vi "GetRFFrame.vi"() -> ()   [LabVIEW 2022 SP3]
uses:
  Motion Controllers/-MotionRoutines/MotionGlobals.vi
  <instrlib>/vi.lib/Platform/portaccess.llb/Out Port32.vi
  <instrlib>/Acqiris Dx/Acqiris Dx.lvlib
  <instrlib>/Acqiris Bx/Acqiris Bx.lvlib
  <instrlib>/niScope/Acquire/Fetch/niScope Multi Fetch Binary 8.vi
  <vilib>/Platform/TimedLoop/XDataNode/XDataNode.xnode
  <vilib>/Platform/TimedLoop/XDataNode/nitl_modes.ctl
  <vilib>/Platform/TimedLoop/XDataNode/XDNodeRunTimeDep.lvlib
  <vilib>/Platform/TimedLoop/XDataNode/wakeup.ctl
  <vilib>/Platform/TimedLoop/XDataNode/timing_clust.ctl
  Pulsers/pulser.ctl
  Acqiris/-AcqirisRoutines/VScaleInfoAcq.vi
panel:
  in  "power":u16(ring)=1 items=["1"=1, "2"=2, "3"=3, "4"=4, "5"=5, "6"=6, "7"=7, "8"=8, "9"=9, "10"=10, "20"=20, "30"=30, "40"=40, "50"=50, "60"=60, "70"=70, "80"=80, "90"=90, "100"=100]
  out "RealFileName":string
  in  "View EYE":bool
  in  "Acq mode":T1(tab)
  in  "Get Frame":bool
  in  "Autosave?":bool
  in  "Save Single":bool
  in  "Reverse Off":bool
  in  "Cont Frame":bool
  in  "Frame Divide":u32=1 min=1
  in  "Fixed Frame Delay":bool
  in  "frame time (ms)":u32=100 min=1
  out "Loop Time":u64=1000
  in  "Total Time (s)":u32=10 min=1
  out "Frame":i32
  in  "Dummy V":dbl
  out "Memory Size (Byte)":i32 format="%^.0e"
  in  "Data Path":path=path "F:/Temp"
  in  "Num of Frames":i32=1
  in  "Set up Dig":bool
  in  "RF cycles":i16=1 min=1
  in  "Display?":bool=TRUE
  in  "ResetNumbing":bool
  in  "file name":string
  out "subarray":i16[][](array[numeric])
  out "Raw data":dbl[][](graph)
  out "Att (dB)":sgl format="%#_1f"
  in  "stop":bool
  in  "Num of Vectors":i32=464
  # "Vevo 770 #s (for header and file name)"
  # "0 dB would scale data to 1 Vpp. 20 dB to 10 Vpp, etc."
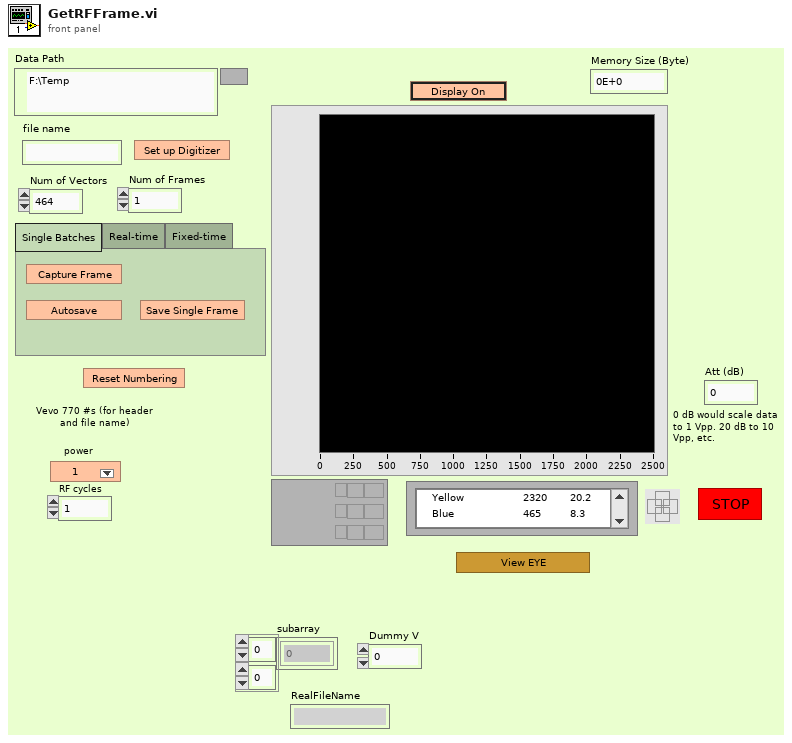
[diagram p1: front panel]
types:
  T1 = enum32{"Single Batches", "Real-time", "Fixed-time"}
  T2 = typedef "pulser.ctl" = enum16{"Pan 5900", "Agilent 33250A", "WMC Mono-Cycle", "Blank", "NYU AVTECH", "Tabor W1281A", "Daxsonics BP1", "Pan 5800", "Daxsonics BP2"}
  T3 = typedef "XDNodeRunTimeDep.lvlib/timing_clust.ctl" = cluster{"Expected End [f-1]":u64, "Actual End [f-1]":u64, "Finished Late? [f-1]":bool, "Expected End [i-1]":u64, "Actual End [i-1]":u64, "Finished Late? [i-1]":bool, "Expected Start [i]":u64, "Actual Start [i]":u64, "Expected Start [f]":u64, "Actual Start [f]":u64, "Source Name":string, "Structure Name":string, "Period":i64, "Deadline":i64, "Offset":i64, "Start":i64, "Priority":i32, "Timeout":i32, "Mode":T4, "Wakeup Reason":T5, "Error":errorcluster, "Source Type":string, "Secondary Source Type":string, "Global End Time":u64, "Global Start Time":u64, "Frame Duration":u64, "Iteration Duration":u64, "Assigned CPU":i32, "I/O Scan Engine Mode":u32}
  T4 = typedef "XDNodeRunTimeDep.lvlib/nitl_modes.ctl" = enum32{"No Change", "Process missed periods, maintain original phase", "Discard missed periods, maintain original phase", "Process missed periods, ignore original phase", "Discard missed periods, ignore original phase"}
  T5 = typedef "XDNodeRunTimeDep.lvlib/wakeup.ctl" = enum32{"Normal", "Aborted", "Asynchronous wakeup", "Timing source error", "Timed loop error", "Timeout"}
  T6 = cluster{"Sampling Rate":dbl, "Ref Delay (ms)":dbl, "rf points per line":i32}
  T7 = cluster{sgl, "Gain [dB]  ":sgl, "Atten (dB)":sgl}
  T8 = cluster{"actualSamples":i32, "absoluteInitialX":dbl, "relativeInitialX":dbl, "xIncrement":dbl, "offset":dbl, "gain":dbl, "reserved1":dbl, "reserved2":dbl}[]
  T9 = cluster{"actualSamples":i32, "absoluteInitialX":dbl, "relativeInitialX":dbl, "xIncrement":dbl, "offset":dbl, "gain":dbl, "reserved1":dbl, "reserved2":dbl}
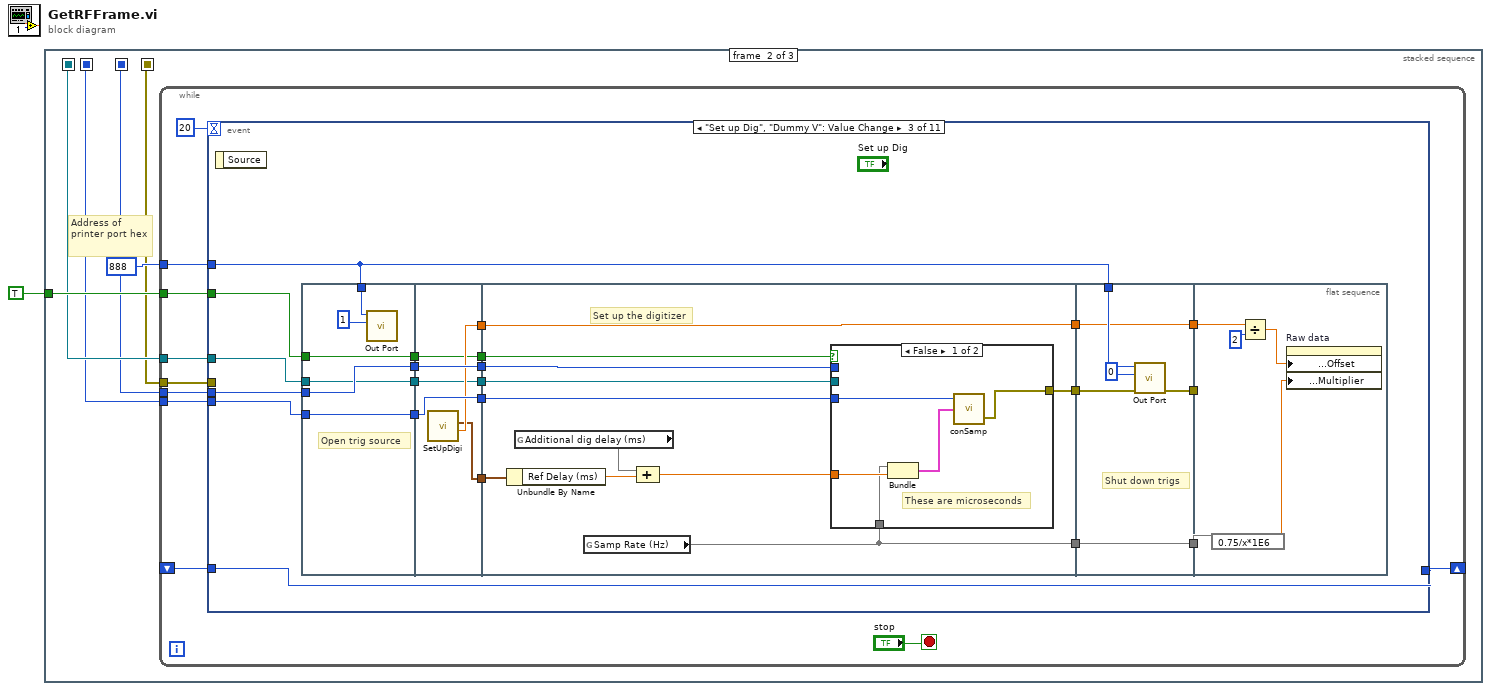
[diagram p0: block diagram]
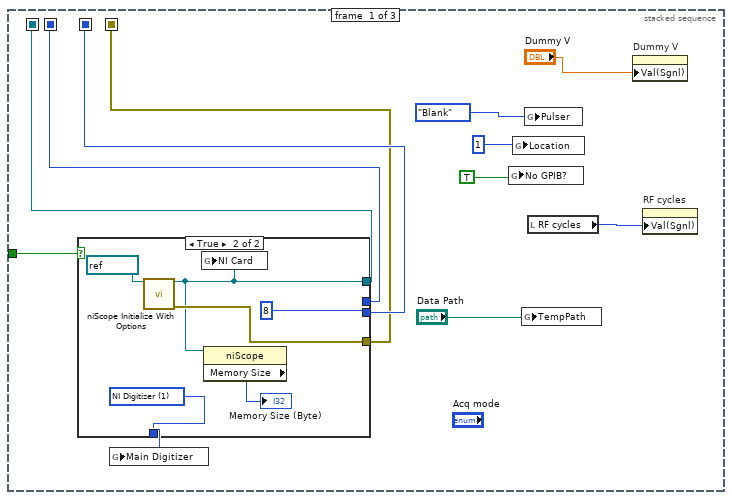
[diagram p2: hidden frame]
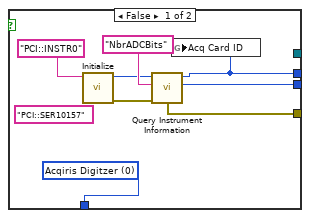
[diagram p3: hidden frame]
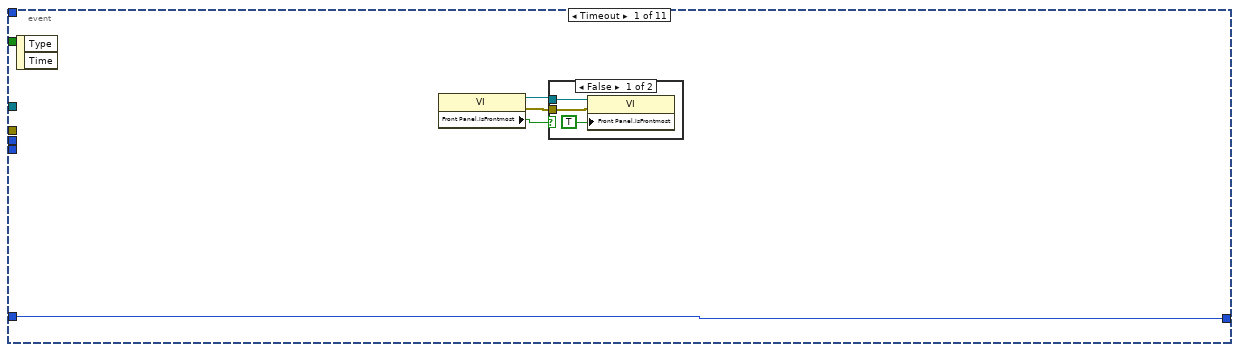
[diagram p4: hidden frame]
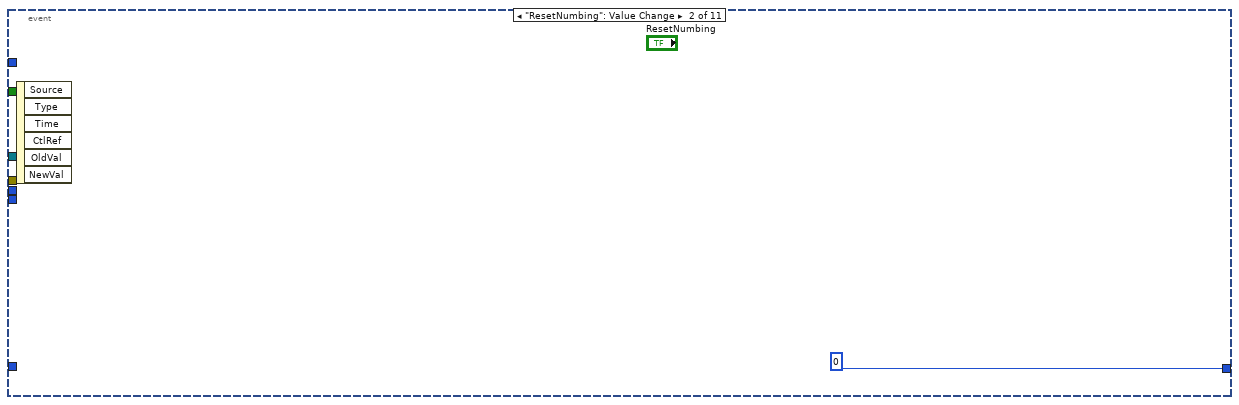
[diagram p6: hidden frame]
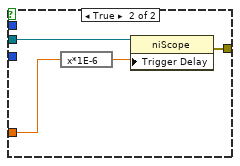
[diagram p7: hidden frame]
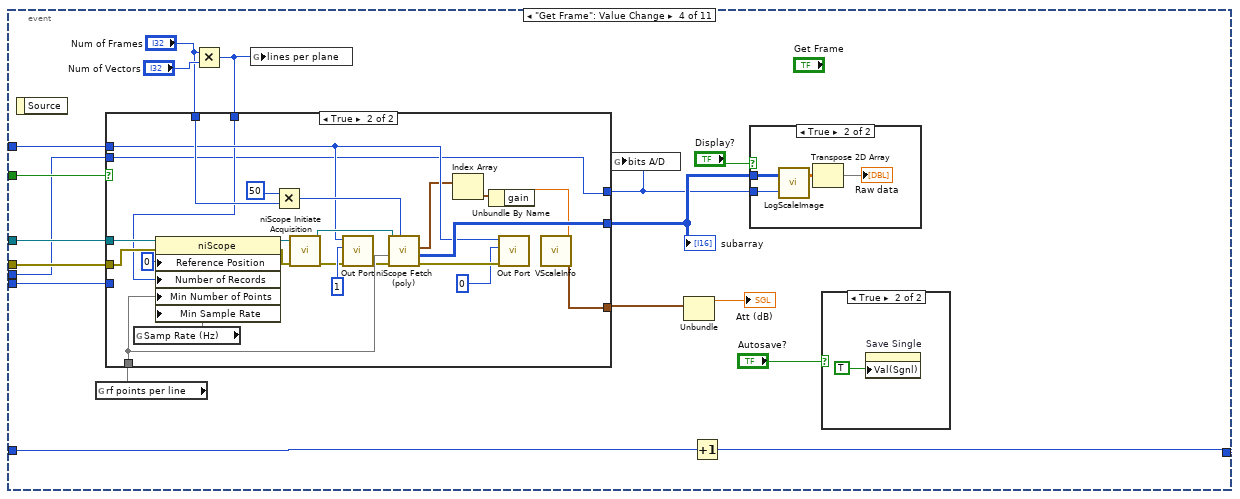
[diagram p8: hidden frame]
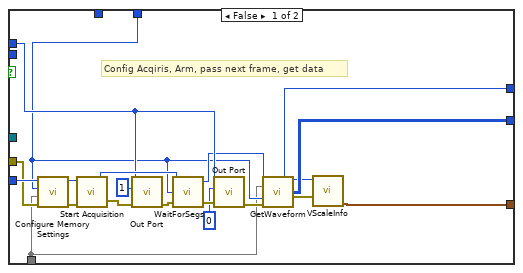
[diagram p9: hidden frame]
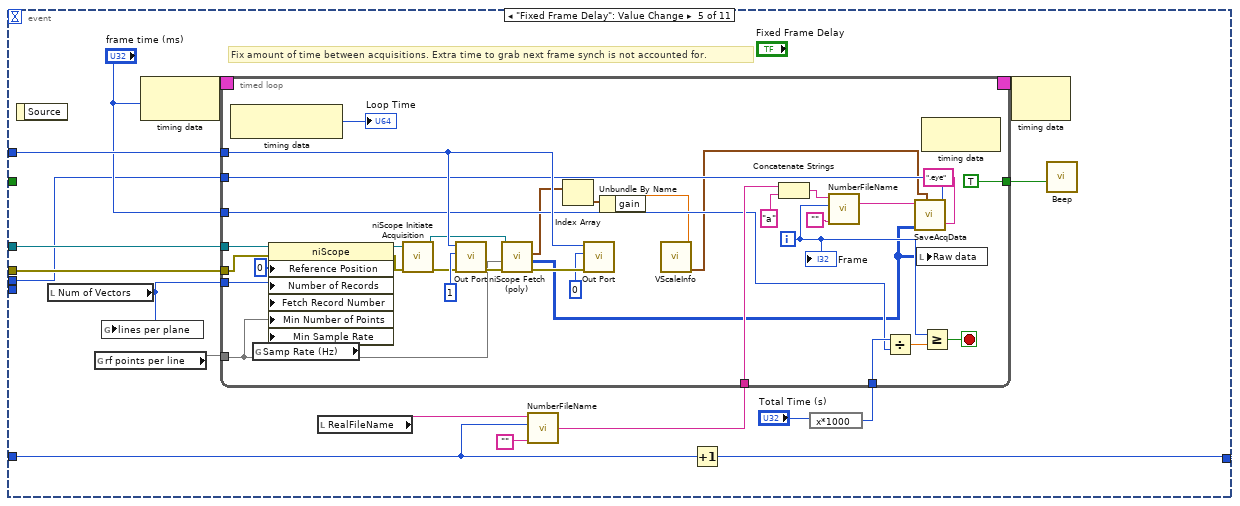
[diagram p12: hidden frame]
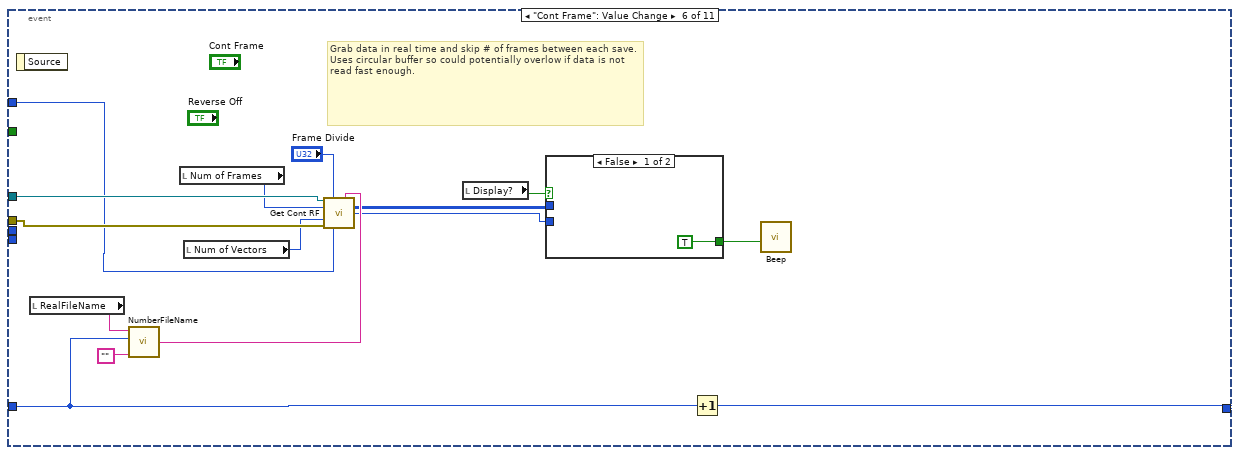
[diagram p13: hidden frame]
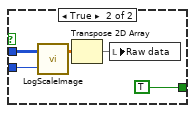
[diagram p14: hidden frame]
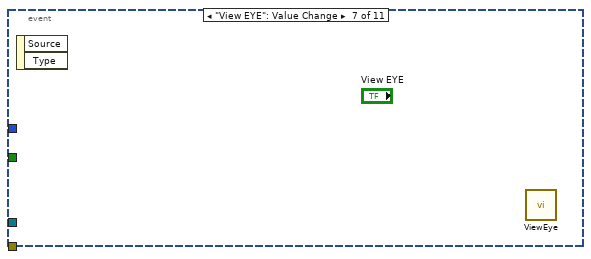
[diagram p15: hidden frame]
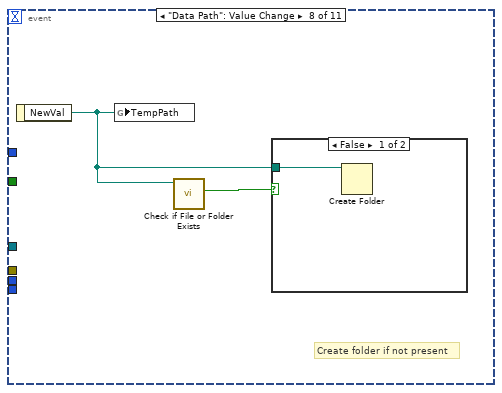
[diagram p16: hidden frame]
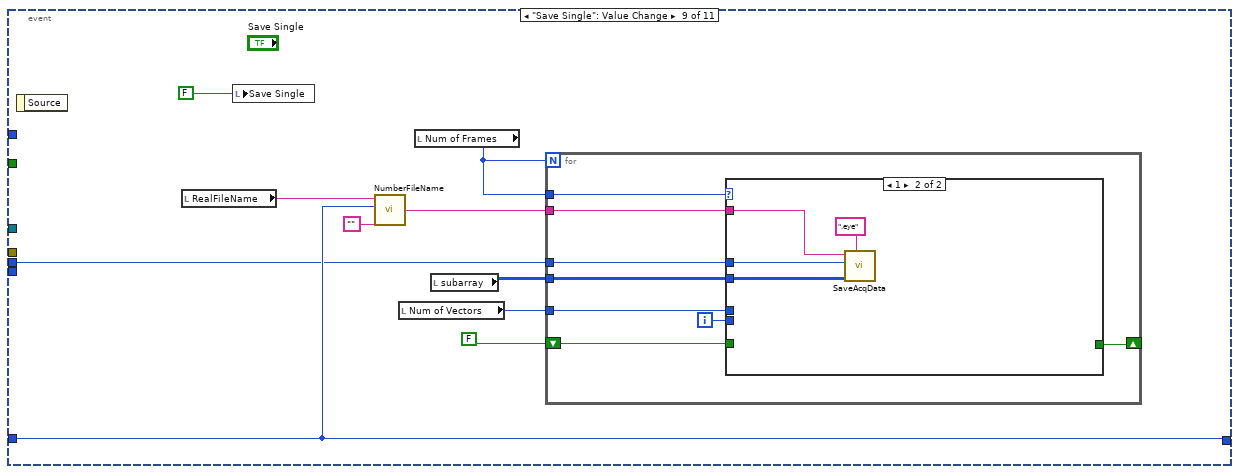
[diagram p18: hidden frame]
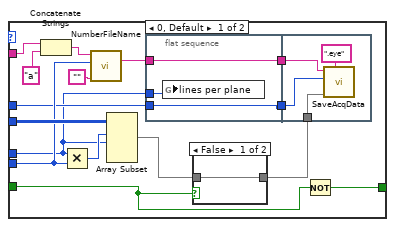
[diagram p19: hidden frame]
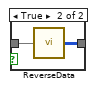
[diagram p20: hidden frame]
diagram:
  n1 = stacked-sequence {
    seq-local: [w9 _ _] -> [_ w31 w320]
    seq-local: [w8 _ _] -> [_ w30 _]
    seq-local: [w7 _ _] -> [_ w29 _]
    seq-local: [w6 _ _] -> [_ w28 _]
    tunnel: TRUE -> [w10 w32 w319]
    frame #0 {
      n2 = case shown="True" w10 {
        tunnel: [_ w24] -> w9
        tunnel: [w18 w25] -> w6
        tunnel: [w14 _] -> w8
        tunnel: [w17 8] -> w7
        tunnel: [w15 w22] -> w11
        frame False {
          w15 = u16 0 items=["Acqiris Digitzer", "NI Digitizer"] ("Main Digitizer")
          (unwired) "PCI::SER10157" ("ResourceName")
          n3 = call <instrlib>:"Initialize.vi"("Resource Name (PCI::INSTR0)"="PCI::INSTR0" ("ResourceName")) -> ("error out"=w19:errorcluster, "Instrument ID"=w20:u32)  [unwired: 3 in, 2 out]
          n4 = call <instrlib>:"Query Instrument Information.vi"("Instrument ID"=w20, "Parameter String"="NbrADCBits", "error in (no error)"=w19) -> ("dup Instrument ID"=w14:u32, "Info Value (I32)"=w17:i32, "error out"=w18:errorcluster)  [unwired: 1 in, 3 out]
          n5 = global write "MotionGlobals.vi" "Acq Card ID"(w14) -> ()
        }
        frame True {
          w22 = u16 1 items=["Acqiris Digitzer", "NI Digitizer"] ("Main Digitizer")
          n6 = call <instrlib>:"niScope Initialize With Options.vi"("resource name"=refnum<k15> "Dig1") -> ("instrument handle"=w24:refnum<k15>, "error out"=w25:errorcluster)  [unwired: 4 in, 9 out]
          n7 = global write "MotionGlobals.vi" "NI Card"(w24) -> ()
          n8 = property class="niScope"(reference=w24) -> ("Memory Size"=→"Memory Size (Byte)":i32)  [unwired: 1 in, 2 out]
        }
      }
      n9 = global write "MotionGlobals.vi" "Main Digitizer"(w11) -> ()
      n10 = global write "MotionGlobals.vi" "No GPIB?"(TRUE ("No GPIB?")) -> ()
      n11 = global write "MotionGlobals.vi" "Location"(1) -> ()
      n12 = global write "MotionGlobals.vi" "TempPath"("Data Path") -> ()
      n13 = global write "MotionGlobals.vi" "Pulser"(pulser."Blank" ("Pulser")) -> ()
      n14 = local read "RF cycles"() -> (w2:i16)
      n15 = property on="Dummy V" class="DigNum (strict)"("Val(Sgnl)"="Dummy V") -> ()  [unwired: 2 in, 2 out]
      n16 = property on="RF cycles" class="DigNum (strict)"("Val(Sgnl)"=w2) -> ()  [unwired: 2 in, 2 out]
    }
    frame #1 {
      # "Address of printer port hex"
      n17 = while {
        tunnel: w31 -> [w43]
        shift-right: [w39] -> _
        shift-left: _ -> [w40]
        tunnel: w30 -> [w38]
        tunnel: w32 -> [w37]
        tunnel: w28 -> [w36]
        tunnel: i16 888 ("address") -> [w35]
        tunnel: w29 -> [w34]
        stop <- "stop" stop-if-true
        n18 = event shown="[2] \"Set up Dig\", \"Dummy V\": Value Change" {
          selector: _ -> [_ _ _ _ _ _ _ _ _ _ _]
          dyn-events: _ -> [_ _ _ _ _ _ _ _ _ _ _]
          timeout: 20 -> [_ _ _ _ _ _ _ _ _ _ _]
          tunnel: w43 -> [_ _ w57 w134 w200 w256 _ _ _ _ _]
          tunnel: w36 -> [_ _ _ w133 w199 w255 _ _ _ _ _]
          tunnel: w40 -> [w47 _ w61 w129 w191 w248 _ _ w275 _ _]
          tunnel: [w47 0 w61 w128 w197 w254 _ _ w275 _ _] -> w39
          tunnel: w38 -> [_ _ w73 w131 _ _ _ _ _ _ _]
          tunnel: w37 -> [_ _ w60 w132 _ _ _ _ _ _ _]
          tunnel: w35 -> [_ _ w72 w130 w198 w251 _ _ _ _ _]
          tunnel: w34 -> [_ _ w71 w117 w184 _ _ _ w274 _ _]
          event Timeout {
            n19 = event-data() -> ()  [unwired: 3 out]
            n20 = property class="VI"() -> (reference out=w46:refnum<vi>, error out=w45:errorcluster, "Front Panel.IsFrontmost"=w44:bool)  [unwired: 2 in]
            n21 = case shown="False" w44 {
              tunnel: w46 -> [w50 _]
              tunnel: w45 -> [w48 _]
              frame False {
                n22 = property class="VI"(reference=w50, error in=w48, "Front Panel.IsFrontmost"=TRUE) -> ()  [unwired: 2 out]
              }
              frame True {
              }
            }
          }
          event "ResetNumbing": Value Change {
            n23 = event-data() -> ()  [unwired: 7 out]
          }
          event "Set up Dig", "Dummy V": Value Change {
            n24 = event-data() -> ()  [unwired: 2 out]
            n25 = flat-sequence {
              tunnel: w73 -> [w79]
              tunnel: [w79] -> w70
              tunnel: w72 -> [w77]
              tunnel: [w76] -> w68
              tunnel: w71 -> [w76]
              tunnel: w60 -> [w75]
              tunnel: [w75] -> w58
              tunnel: w57 -> [w74]
              tunnel: [w74] -> w55
              tunnel: w70 -> [w84]
              tunnel: [w84] -> w69
              tunnel: w68 -> [w85]
              tunnel: [w85] -> w67
              tunnel: [w83] -> w62
              tunnel: [w82] -> w59
              tunnel: w58 -> [w82]
              tunnel: [w81] -> w56
              tunnel: w55 -> [w81]
              tunnel: [w80] -> w54
              tunnel: w69 -> [w96]
              tunnel: w67 -> [w95]
              tunnel: [w87] -> w65
              tunnel: [w86] -> w63
              tunnel: w62 -> [w86]
              tunnel: w59 -> [w94]
              tunnel: w56 -> [w93]
              tunnel: w54 -> [w92]
              tunnel: [w88] -> w53
              tunnel: w72 -> [w110]
              tunnel: [w109] -> w66
              tunnel: w65 -> [w109]
              tunnel: [w108] -> w64
              tunnel: w63 -> [w108]
              tunnel: w53 -> [w107]
              tunnel: [w106] -> w52
              tunnel: w66 -> [w116]
              tunnel: w64 -> [w113]
              tunnel: w52 -> [_]
              frame #0 {
                # "Open trig source"
                n26 = call-poly <instrlib>:"Out Port.vi"("write value"=1, "address"=w77) -> ()  [unwired: 1 in, 7 out]
              }
              frame #1 {
                n27 = call "SetUpDigi.vi"() -> ("Equivalent RT delay\ndistance (mm)"=w83:dbl, "RF data Sampling Out"=w80:T6)  [unwired: 5 in, 5 out]
              }
              frame #2 {
                # "Set up the digitizer"
                n28 = Unbundle By Name(w92) -> ("Ref Delay (ms)"=w90:dbl)
                n29 = global read "MotionGlobals.vi" "Additional dig delay (ms)"() -> (w91)
                n30 = global read "MotionGlobals.vi" "Samp Rate (Hz)"() -> (w87)
                n31 = Compound Arithmetic op=ADD(w91, w90) -> (w89:dbl)
                n32 = case shown="False" w94 {
                  tunnel: w96 -> [w98 _]
                  tunnel: w95 -> [_ _]
                  tunnel: w93 -> [_ w102]
                  tunnel: w89 -> [w101 w104]
                  tunnel: [w99 w103] -> w88
                  tunnel: w87 -> [w97 _]
                  frame False {
                    # "These are microseconds"
                    n33 = Bundle("Samp Rate (Hz)"=w97, w101) -> (w100:cluster{"Samp Rate (Hz)":void, dbl})  [unwired: 1 out]
                    n34 = call "conSamp.vi"("Sampling"=w100, "InstrumentID"=w98) -> ("error out"=w99:errorcluster)  [unwired: 1 in, 1 out]
                  }
                  frame True {
                    n35 = expression code="x*1E-6"(w104) -> (w105:dbl)
                    n36 = property class="niScope"(reference=w102, "Trigger Delay"=w105) -> (error out=w103:errorcluster)  [unwired: 1 in, 1 out]
                  }
                }
              }
              frame #3 {
                # "Shut down trigs"
                n37 = call-poly <instrlib>:"Out Port.vi"("error in (no error)"=w107, "write value"=0, "address"=w110) -> ("error out"=w106:errorcluster)  [unwired: 6 out]
              }
              frame #4 {
                n38 = expression code="0.75/x*1E6"(w116) -> (w115:dbl)
                n39 = Divide(x=w113, y=2) -> (x/y=w112:dbl)
                n40 = property on="Raw data" class="IntGraph (strict)"("Y Scale.Offset and Multiplier:Offset"=w112, "Y Scale.Offset and Multiplier:Multiplier"=w115) -> ()  [unwired: 2 in, 2 out]
              }
            }
          }
          event "Get Frame": Value Change {
            n41 = event-data() -> ()  [unwired: 2 out]
            n42 = global read "MotionGlobals.vi" "rf points per line"() -> (w125)
            n43 = Multiply(x="Num of Frames", y="Num of Vectors") -> (x*y=w124:i32)
            n44 = case shown="True" w132 {
              tunnel: w134 -> [_ w173]
              tunnel: w133 -> [w151 w172]
              tunnel: [w142 w177] -> w121
              tunnel: [w137 w158] -> w119
              tunnel: w131 -> [w154 _]
              tunnel: w130 -> [w146 w163]
              tunnel: w124 -> [w136 w161]
              tunnel: w125 -> [w135 w171]
              tunnel: [w143 w176] -> w118
              tunnel: "Num of Frames" -> [_ w168]
              tunnel: w117 -> [_ w158]
              frame False {
                # "Config Acqiris, Arm, pass next frame, get data"
                n45 = call <instrlib>:"Configure Memory Settings.vi"("error in (no error)"=w151, "Number of Samples (1000)"=w135, "Number of Segments (1)"=w136, "Instrument ID"=w154) -> ("error out"=w152:errorcluster, "dup Instrument ID"=w153:u32)  [unwired: 2 out]
                n46 = call <instrlib>:"Start Acquisition.vi"("error in (no error)"=w152, "Instrument ID"=w153) -> ("error out"=w148:errorcluster, "dup Instrument ID"=w150:u32)  [unwired: 2 in]
                n47 = call-poly <instrlib>:"Out Port.vi"("error in (no error)"=w148, "write value"=1, "address"=w146) -> ("error out"=w147:errorcluster)  [unwired: 6 out]
                n48 = call "WaitForSegs.vi"("Acqiris ID"=w150, "lines per plane"=w136, "error in"=w147) -> ("dup Instrument ID"=w141:u32, "error out"=w149:errorcluster)  [unwired: 1 in, 2 out]
                n49 = call-poly <instrlib>:"Out Port.vi"("error in (no error)"=w149, "write value"=0, "address"=w146) -> ("error out"=w138:errorcluster)  [unwired: 6 out]
                n50 = call "GetWaveform.vi"("Acq ID Out"=w141, "Num Samps"=w135, "Num Segs"=w136, "error in"=w138) -> ("Dig Word Size"=w137:u16, "Acq ID Out"=w140:u32, "Acquired Waveform16 bit"=w142:i16[][], "error out"=w139:errorcluster)  [unwired: 2 in, 6 out]
                n51 = call-poly "VScaleInfo.vi"(4:w139, "vGain scalar"=w140) -> ("Voltage Scale"=w143:T7)  [unwired: 6 in, 2 out]
              }
              frame True {
                n52 = global read "MotionGlobals.vi" "Samp Rate (Hz)"() -> (w159)
                n53 = property class="niScope"(reference=w173, error in=w172, "Reference Position"=0, "Number of Records"=w161, "Min Number of Points"=w171, "Min Sample Rate"=w159) -> (reference out=w175:refnum<k15>, error out=w174:errorcluster)
                n54 = Multiply(x=50, y=w168) -> (x*y=w169:i32)
                n55 = call <instrlib>:"niScope Initiate Acquisition.vi"("instrument handle"=w175, "error in"=w174) -> ("instrument handle out"=w178:refnum<k15>, "error out"=w166:errorcluster)  [unwired: 12 out]
                n56 = call-poly <instrlib>:"Out Port.vi"("error in (no error)"=w166, "write value"=1, "address"=w163) -> ("error out"=w165:errorcluster)  [unwired: 6 out]
                n57 = call-poly <instrlib>:"niScope Fetch (poly).vi"("timeout"=w169, "error in"=w165, "numSamples"=w171, "instrument handle"=w178) -> ("error out"=w164:errorcluster, "wfm"=w177:i8[][], "wfm info"=w157:T8)  [unwired: 1 in, 4 out]
                n58 = Index Array(array=w157) -> (element=w156:T9)  [unwired: 1 in]
                n59 = Unbundle By Name(w156) -> ("gain"=w155:dbl)
                n60 = call-poly <instrlib>:"Out Port.vi"("error in (no error)"=w164, "write value"=0, "address"=w163) -> ()  [unwired: 7 out]
                n61 = call-poly "VScaleInfo.vi"("vGain scalar"=w155) -> ("Voltage Scale"=w176:T7)  [unwired: 7 in, 2 out]
              }
            }
            "subarray" <- w121
            n62 = global write "MotionGlobals.vi" "lines per plane"(w124) -> ()
            n63 = global write "MotionGlobals.vi" "bits A/D"(w119) -> ()
            n64 = Unbundle(w118) -> (→"Att (dB)":sgl)  [unwired: 2 out]
            n65 = Increment(x=w129) -> (x+1=w128:i32)
            n66 = case shown="True" "Display?" {
              tunnel: w121 -> [_ w182]
              tunnel: w119 -> [_ w180]
              frame False {
              }
              frame True {
                n67 = call "LogScaleImage.vi"("A/D bits"=w180, "input array"=w182) -> ("log scale image"=w181:dbl[][])  [unwired: 1 out]
                n68 = Transpose 2D Array(2D array=w181) -> (transposed array=→"Raw data":dbl[][])
              }
            }
            n69 = case shown="True" "Autosave?" {
              frame False {
              }
              frame True {
                n70 = property on="Save Single" class="Bool (strict)"("Val(Sgnl)"=TRUE ("Value (Signaling)")) -> ()  [unwired: 2 in, 2 out]
              }
            }
          }
          event "Fixed Frame Delay": Value Change {
            # "Fix amount of time between acquisitions. Extra time to grab next frame synch is not accounted for."
            n71 = event-data() -> ()  [unwired: 2 out]
            n72 = local read "Num of Vectors"() -> (w195:i32)
            n73 = global read "MotionGlobals.vi" "rf points per line"() -> (w196)
            n74 = global write "MotionGlobals.vi" "lines per plane"(w195) -> ()
            n75 = node-c288("frame time (ms)") -> (w194:T3)
            n76 = local read "RealFileName"() -> (w192:string)
            n77 = call "NumberFileName.vi"("String"="", "File number"=w191, "file name"=w192) -> ("Numbered File"=w189:string)  [unwired: 1 in]
            n78 = Increment(x=w191) -> (x+1=w197:i32)
            n79 = expression code="x*1000"("Total Time (s)") -> (w187:u32)
            n80 = timed-loop {
              timing: w194 -> [_]
              timing-out: [_] -> w193
              tunnel: w200 -> [w234]
              tunnel: w199 -> [w233]
              tunnel: w198 -> [w232]
              tunnel: w196 -> [w214]
              tunnel: w195 -> [w222]
              tunnel: w189 -> [w217]
              tunnel: w187 -> [w213]
              tunnel: "frame time (ms)" -> [w212]
              tunnel: [TRUE] -> w185
              tunnel: w184 -> [w205]
              i -> [w211]
              stop <- w209 stop-if-true
              w208 = 0
              n81 = node-c288() -> (→"Loop Time":i64)  [unwired: 1 out]
              n82 = global read "MotionGlobals.vi" "Samp Rate (Hz)"() -> (w223)
              n83 = property class="niScope"(reference=w234, error in=w233, "Reference Position"=w208, "Number of Records"=w222, "Fetch Record Number"=w208, "Min Number of Points"=w214, "Min Sample Rate"=w223) -> (reference out=w230:refnum<k15>, error out=w229:errorcluster)
              n84 = call <instrlib>:"niScope Initiate Acquisition.vi"("instrument handle"=w230, "error in"=w229) -> ("instrument handle out"=w231:refnum<k15>, "error out"=w227:errorcluster)  [unwired: 12 out]
              n85 = call-poly <instrlib>:"Out Port.vi"("error in (no error)"=w227, "write value"=1, "address"=w232) -> ("error out"=w226:errorcluster)  [unwired: 6 out]
              n86 = call-poly <instrlib>:"niScope Fetch (poly).vi"("error in"=w226, "numSamples"=w214, "instrument handle"=w231) -> ("error out"=w225:errorcluster, "wfm"=w207:i8[][], "wfm info"=w203:T8)  [unwired: 2 in, 4 out]
              n87 = Index Array(array=w203) -> (element=w202:T9)  [unwired: 1 in]
              n88 = call-poly <instrlib>:"Out Port.vi"("error in (no error)"=w225, "write value"=0, "address"=w232) -> ()  [unwired: 7 out]
              n89 = Unbundle By Name(w202) -> ("gain"=w201:dbl)
              n90 = call-poly "VScaleInfo.vi"("vGain scalar"=w201) -> ("Voltage Scale"=w204:T7)  [unwired: 7 in, 2 out]
              n91 = Concatenate Strings(w217, "a") -> (w220:string)
              n92 = call "NumberFileName.vi"("String"="", "File number"=w211, "file name"=w220) -> ("Numbered File"=w219:string)  [unwired: 1 in]
              n93 = Divide(x=w213, y=w212) -> (x/y=w210:dbl)
              n94 = call "SaveAcqData.vi"("Ext"=".eye", "Votage scaling"=w204, "Array"=w207, "Dig Word Size"=w205, "File Name"=w219) -> ()  [unwired: 2 in]
              n95 = local write "Raw data"(w207) -> ()
              n96 = node-c288() -> ()  [unwired: 2 out]
              n97 = Greater Or Equal?(x=w211, y=w210) -> (x >= y?=w209:bool)
              "Frame" <- w211
            }
            n98 = node-c288(w193) -> ()  [unwired: 1 out]
            n99 = call <vilib>:"Beep.vi"("use system alert? (T)"=w185) -> ()  [unwired: 2 in, 9 out]
          }
          event "Cont Frame": Value Change {
            # "Grab data in real time and skip # of frames between each save. Uses circular buffer so could potentially overlow if data is not read fast enough."
            n100 = event-data() -> ()  [unwired: 2 out]
            n101 = local read "RealFileName"() -> (w242:string)
            n102 = call "NumberFileName.vi"("String"="", "File number"=w248, "file name"=w242) -> ("Numbered File"=w247:string)  [unwired: 1 in]
            n103 = local read "Num of Frames"() -> (w253:i32)
            n104 = local read "Num of Vectors"() -> (w252:i32)
            n105 = call "Get Cont RF.vi"("instrument handle"=w256, "Skip Frames"="Frame Divide", "file name"=w247, "Num of Frames"=w253, "Num of Vectors"=w252, "error out"=w255, "address"=w251) -> ("Array out"=w246:i8[][], "Dig Word Size"=w245:u16)  [unwired: 1 in, 6 out]
            n106 = local read "Display?"() -> (w244:bool)
            n107 = case shown="False" w244 {
              tunnel: w246 -> [_ w262]
              tunnel: w245 -> [_ w260]
              tunnel: [TRUE TRUE] -> w243
              frame False {
              }
              frame True {
                n108 = call "LogScaleImage.vi"("A/D bits"=w260, "input array"=w262) -> ("log scale image"=w261:dbl[][])  [unwired: 1 out]
                n109 = Transpose 2D Array(2D array=w261) -> (transposed array=w259:dbl[][])
                n110 = local write "Raw data"(w259) -> ()
              }
            }
            n111 = Increment(x=w248) -> (x+1=w254:i32)
            n112 = call <vilib>:"Beep.vi"("use system alert? (T)"=w243) -> ()  [unwired: 2 in, 9 out]
          }
          event "View EYE": Value Change {
            n113 = event-data() -> ()  [unwired: 3 out]
            n114 = call "ViewEye.vi"() -> ()  [unwired: 1 out]
          }
          event "Data Path": Value Change {
            # "Create folder if not present"
            n115 = event-data() -> ("NewVal"=w263:path)  [unwired: 1 out]
            n116 = global write "MotionGlobals.vi" "TempPath"(w263) -> ()
            n117 = call <vilib>:"Check if File or Folder Exists.vi"("path"=w263) -> ("file or folder exists?"=w264:bool)  [unwired: 1 in, 9 out]
            n118 = case shown="False" w264 {
              tunnel: w263 -> [w265 _]
              frame False {
                n119 = Create Folder(path (use dialog)=w265) -> ()  [unwired: 1 in, 4 out]
              }
              frame True {
              }
            }
          }
          event "Save Single": Value Change {
            n120 = event-data() -> ()  [unwired: 2 out]
            n121 = local read "RealFileName"() -> (w266:string)
            n122 = local write "Save Single"(FALSE) -> ()
            n123 = call "NumberFileName.vi"("String"="", "File number"=w275, "file name"=w266) -> ("Numbered File"=w271:string)  [unwired: 1 in]
            n124 = local read "Num of Vectors"() -> (w270:i32)
            n125 = local read "Num of Frames"() -> (w269:i32)
            n126 = local read "subarray"() -> (w272:i16[][])
            n127 = for {
              N: w269 -> [_]
              tunnel: w272 -> [w283]
              tunnel: w274 -> [w282]
              tunnel: w271 -> [w281]
              tunnel: w269 -> [w280]
              tunnel: w270 -> [w278]
              shift-right: [w276] -> _
              shift-left: FALSE -> [w277]
              i -> [w279]
              n128 = case shown="1" w280 {
                tunnel: w283 -> [w299 w313]
                tunnel: w282 -> [w288 w312]
                tunnel: w281 -> [w287 w311]
                tunnel: w279 -> [w297 _]
                tunnel: w278 -> [w284 _]
                tunnel: w277 -> [w293 _]
                tunnel: [w295 _] -> w276
                frame 0, Default {
                  n129 = Concatenate Strings(w287, "a") -> (w286:string)
                  n130 = Multiply(x=w284, y=w297) -> (x*y=w298:i32)
                  n131 = call "NumberFileName.vi"("String"="", "File number"=w297, "file name"=w286) -> ("Numbered File"=w290:string)  [unwired: 1 in]
                  n132 = Array Subset(array=w299, index (row)=w298, length (row)=w284) -> (w292:i16[][])  [unwired: 2 in]
                  n133 = flat-sequence {
                    tunnel: [w305] -> w291
                    tunnel: w290 -> [w305]
                    tunnel: [w304] -> w289
                    tunnel: w288 -> [w304]
                    tunnel: w284 -> [w303]
                    tunnel: w294 -> [w309]
                    tunnel: w291 -> [w308]
                    tunnel: w289 -> [w307]
                    frame #0 {
                      n134 = global write "MotionGlobals.vi" "lines per plane"(w303) -> ()
                    }
                    frame #1 {
                      n135 = call "SaveAcqData.vi"("Ext"=".eye", "Array"=w309, "Dig Word Size"=w307, "File Name"=w308) -> ()  [unwired: 3 in]
                    }
                  }
                  n136 = case shown="False" w293 {
                    tunnel: [w300 w302] -> w294
                    tunnel: w292 -> [w300 w301]
                    frame False {
                    }
                    frame True {
                      n137 = call "ReverseData.vi"("Array in"=w301) -> ("Array out"=w302:i16[][])
                    }
                  }
                  n138 = Not(x=w293) -> (.not. x?=w295:bool)
                }
                frame 1 {
                  n139 = call "SaveAcqData.vi"("Ext"=".eye", "Array"=w313, "Dig Word Size"=w312, "File Name"=w311) -> ()  [unwired: 3 in]
                }
              }
            }
          }
          event "Frame Divide": Value Change {
            n140 = event-data() -> ("NewVal"=w314:u32)  [unwired: 1 out]
            n141 = global write "MotionGlobals.vi" "F Zones"(w314) -> ()
          }
          event "file name", "power", "RF cycles": Value Change {
            n142 = event-data() -> ()  [unwired: 2 out]
            n143 = global write "MotionGlobals.vi" "power"("power") -> ()
            n144 = global write "MotionGlobals.vi" "RF cycles"("RF cycles") -> ()
            n145 = call "Build Text"("Beginning Text"="file name", "p"="power", "rf"="RF cycles") -> ("Result"=→"RealFileName":string)  [unwired: 11 in, 1 out]
          }
        }
      }
    }
    frame #2 {
      n146 = case shown="True" w319 {
        tunnel: w320 -> [_ w321]
        frame False {
        }
        frame True {
          n147 = call <instrlib>:"niScope Close.vi"("instrument handle"=w321) -> ()  [unwired: 1 in, 14 out]
        }
      }
    }
  }
